vi "_PC_Err write_error_message.vi"(5 "skipWrong( T )":bool=TRUE, 7 "show msg( T )":bool=TRUE, 8 "error in":errorcluster) -> (0 "error out":errorcluster)   [LabVIEW 2018]
uses:
  Constant/AccessFolderName.ctl
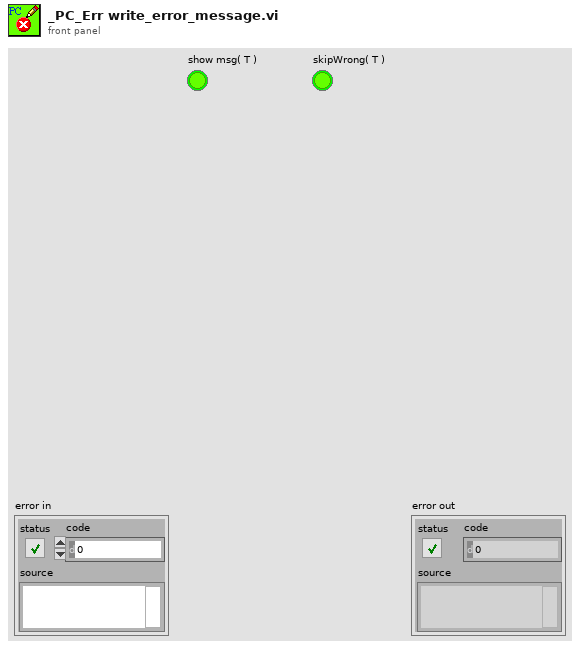
[diagram p1: front panel]
types:
  T1 = typedef "AccessFolderName.ctl" = enum16{"None", "system_log", "ui_log", "msdata", "method", "d999_param"}
  T2 = enum16{"open", "replace", "create", "open or create", "replace or create", "replace or create with confirmation"}
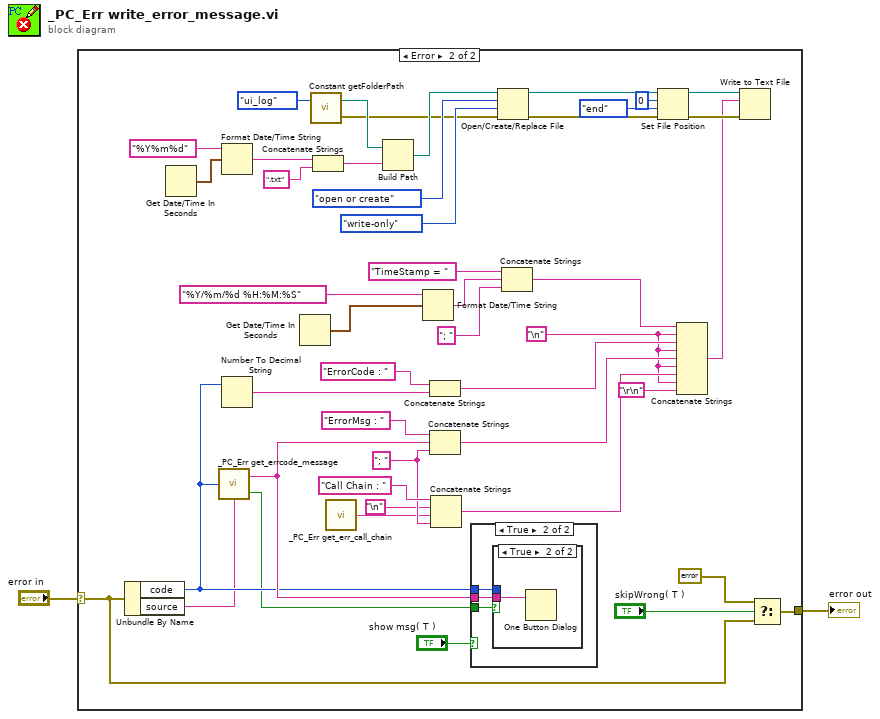
[diagram p0: block diagram]
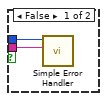
[diagram p4: hidden frame]
diagram:
  n1 = case shown="Error" "error in" {
    selector: "error in" -> [w3 w8]
    tunnel: [w3 w6] -> w1
    frame No Error {
    }
    frame Error {
      w13 = "\n"
      w16 = "; " ("string")
      n2 = Unbundle By Name(w8) -> ("code"=w10:i32, "source"=w5:string)
      n3 = Get Date/Time In Seconds() -> (seconds since 1Jan1904=w48:timestamp)
      n4 = call "_PC_Err get_errcode_message.vi"("err code"=w10, "sourceError"=w5) -> ("err msg"=w11:string, "customError"=w4:bool)
      n5 = Format Date/Time String(time format string (%c)="%Y%m%d", seconds (now)=w48) -> (date/time string=w46:string)  [unwired: 1 in]
      n6 = Number To Decimal String(number=w10) -> (decimal integer string=w25:string)  [unwired: 1 in]
      n7 = Get Date/Time In Seconds() -> (seconds since 1Jan1904=w31:timestamp)
      n8 = call "Constant getFolderPath.vi"("folder name"=AccessFolderName."ui_log") -> ("error out"=w20:errorcluster, "folder path"=w21:path)  [unwired: 1 in]
      n9 = Concatenate Strings(w46, ".txt" ("string")) -> (w44:string)
      n10 = call "_PC_Err get_err_call_chain.vi"() -> ("call chain string"=w14:string)
      n11 = Build Path(base path=w21, name or relative path=w44) -> (appended path=w43:path)
      n12 = Format Date/Time String(time format string (%c)="%Y/%m/%d %H:%M:%S", seconds (now)=w31) -> (date/time string=w32:string)  [unwired: 1 in]
      n13 = Concatenate Strings("ErrorCode : " ("string"), w25) -> (w23:string)
      n14 = Concatenate Strings("ErrorMsg : " ("string"), w11, w16) -> (w24:string)
      n15 = Concatenate Strings("Call Chain : " ("string"), "\n", w14, w16) -> (w17:string)
      n16 = case shown="True" "show msg( T )" {
        tunnel: w11 -> [_ w50]
        tunnel: w10 -> [_ w51]
        tunnel: w4 -> [_ w49]
        frame False {
        }
        frame True {
          n17 = case shown="True" w49 {
            tunnel: w51 -> [w53 _]
            tunnel: w50 -> [w52 w54]
            frame False {
              n18 = call <vilib>:"Simple Error Handler.vi"("error code (no error:0)"=w53, "error source (\" \")"=w52) -> ()  [unwired: 3 in, 5 out]
            }
            frame True {
              n19 = One Button Dialog(message=w54) -> ()  [unwired: 1 in, 1 out]
            }
          }
        }
      }
      n20 = Open/Create/Replace File(file path (use dialog)=w43, error in=w20, operation (0:open)=T2."open or create", access (0:read/write)=enum16{"read/write", "read-only", "write-only"}."write-only") -> (refnum out=w36:refnum<file>, error out=w35:errorcluster)  [unwired: 2 in, 1 out]
      n21 = Concatenate Strings("TimeStamp = " ("string"), w32, "; " ("string")) -> (w19:string)
      n22 = Set File Position(offset (in bytes) (0)=i64 0, refnum=w36, from (0:start)=enum16{"start", "end", "current"}."end", error in=w35) -> (refnum out=w38:refnum<file>, error out=w37:errorcluster)
      n23 = Concatenate Strings(w19, w13, w23, w13, w24, w13, w17, w13, "\r\n") -> (w34:string)
      n24 = Write to Text File(file (use dialog)=w38, text=w34, error in=w37) -> ()  [unwired: 1 in, 3 out]
      n25 = Select(t=errorcluster {"status"=FALSE, "code"=0, "source"=""}, s="skipWrong( T )", f=w8) -> (s? t:f=w6:errorcluster)
    }
  }
  "error out" <- w1
